vi "Set_Sequence_Step_Numbers.vi"(1 "Input Sequence":cluster{string, string[], dbl[], dbl}[](array[cluster])) -> (0 "Output Sequence":cluster{string, string[], dbl[], dbl}[](array[cluster]))   [LabVIEW 2011]
doc: "This VI iterates through a sequence and sets a parameter designating each command's placement in the sequence. For example, 14/20."
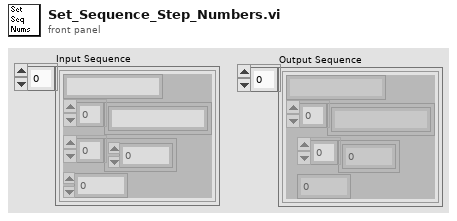
[diagram p1: front panel]
types:
  T1 = cluster{string, "Argument List Out":string[], dbl[], dbl}
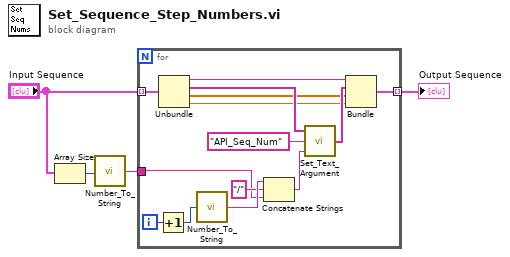
[diagram p0: block diagram]
diagram:
  n1 = Array Size(array="Input Sequence") -> (size(s)=w2:i32)
  n2 = call "Number_To_String.vi"("Number"=w2) -> ("String"=w1:string)
  n3 = for {
    tunnel: "Input Sequence" -> [w17] mode=indexing
    tunnel: [w15] -> w4 mode=indexing
    tunnel: w1 -> [w8]
    i -> [w6]
    n4 = Increment(x=w6) -> (x+1=w5:i32)
    n5 = Unbundle(w17) -> (w14:string, w16:string[], w12:dbl[], w11:dbl)
    n6 = call "Number_To_String.vi"("Number"=w5) -> ("String"=w10:string)
    n7 = Concatenate Strings(w10, "/" ("string"), w8) -> (w7:string)
    n8 = call "Set_Text_Argument.vi"("Text"=w7, "Argument"="API_Seq_Num", "Argument List In"=w16) -> ("Argument List Out"=w13:string[])
    n9 = Bundle(w14, "Argument List Out"=w13, w12, w11) -> (w15:T1)  [unwired: 1 in]
  }
  "Output Sequence" <- w4
